vi "DSF.Shared.Timing.Get Decimation.vi"(11 "Timing in":refnum<class "DSF.Shared.Timing.lvclass">) -> (2 "Decimation":T1=1, 3 "Timing out":refnum<class "DSF.Shared.Timing.lvclass">)   [LabVIEW 2017, in "DSF.Shared.lvlib" / "DSF.Shared.Timing.lvclass"]
uses:
  DSF.Shared.Timing.lvclass
  Typedefs/DSF.Shared.Typedefs.Scalars.Decimation.ctl
  DSF.Shared.Timing.lvclass/DSF.Shared.Timing.ctl
  DSF.Shared.lvlib
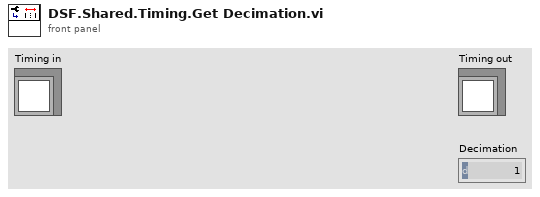
[diagram p1: front panel]
types:
  T1 = typedef "DSF.Shared.lvlib/DSF.Shared.Typedefs.Scalars.Decimation.ctl" = u64
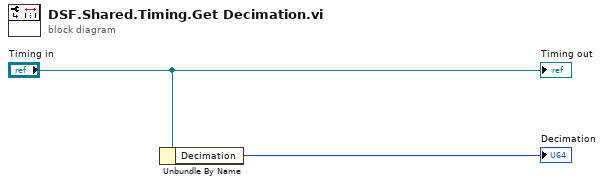
[diagram p0: block diagram]
diagram:
  n1 = Unbundle By Name("Timing in") -> ("Decimation"=→"Decimation":T1)
  "Timing out" <- "Timing in"
